vi "Write Value.vi"(8 "error in (no error)":errorcluster, 10 "Value":waveform(dbl), 11 "Const_WFM in":refnum<class "Const_WFM.lvclass">) -> (0 "error out":errorcluster, 3 "Const_WFM out":refnum<class "Const_WFM.lvclass">)   [LabVIEW 2021, in "Const_WFM.lvclass"]
uses:
  Const_WFM.lvclass
  Const_WFM.lvclass/Const_WFM.ctl
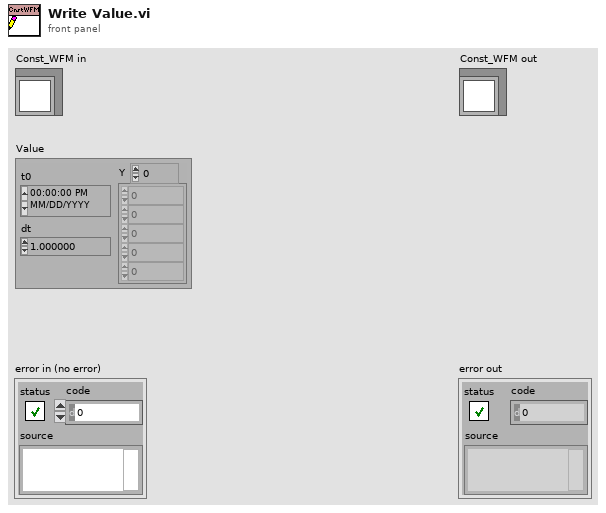
[diagram p1: front panel]
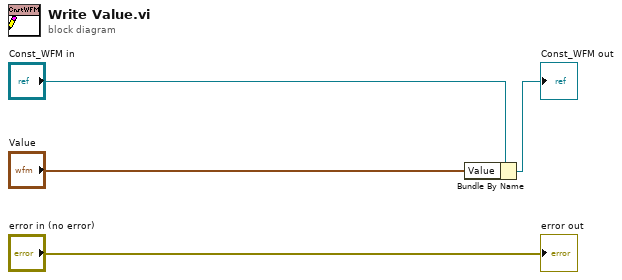
[diagram p0: block diagram]
diagram:
  n1 = Bundle By Name(cluster="Const_WFM in", "Value"="Value") -> (→"Const_WFM out":refnum<class "Const_WFM.lvclass">)
  "error out" <- "error in (no error)"
